vi "terminal point.vi"(2 "peaks/valleys":enum32{"Peaks", "Valleys"}(ring)=enum."Valleys", 3 "threshold":dbl caption="阈值" format="%0.2f", 4 "PD width":i32=3 caption="PD宽度" min=3, 5 "TDD filePath":path caption="TDD file Path") -> (0 "time low":dbl, 1 "time low index":dbl)   [LabVIEW 2011]
uses:
  <vilib>/Utility/file.llb/Read From Spreadsheet File (DBL).vi
  <vilib>/Analysis/NI_AAL_SigProc.lvlib
panel:
  out "XY图":cluster{"all rows":dbl[], "all rows":dbl[]}[](graph)
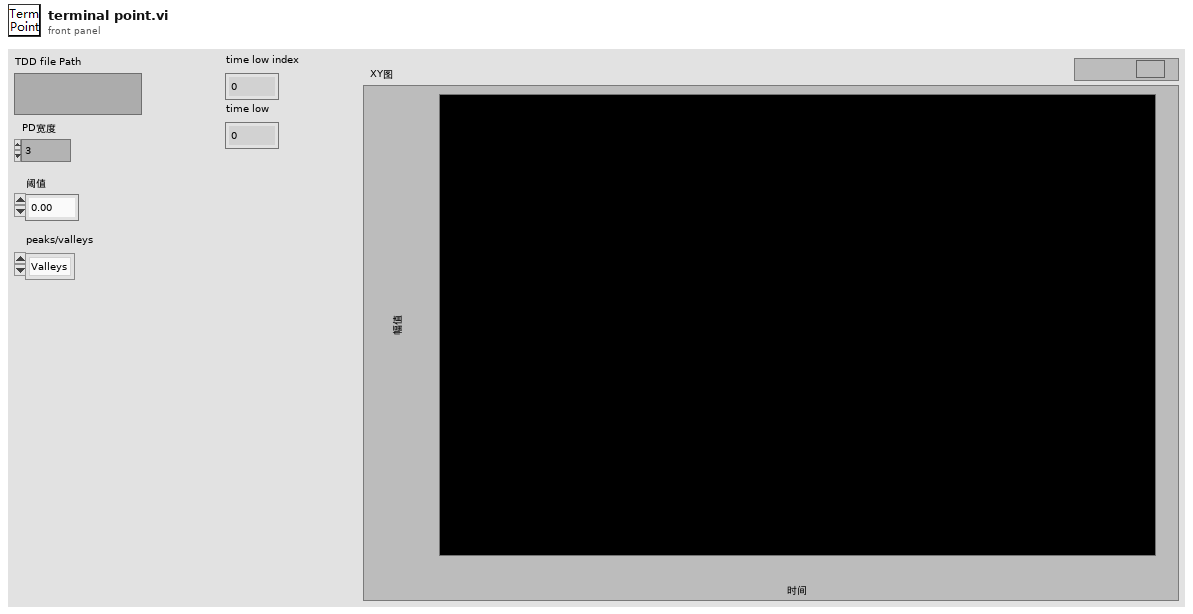
[diagram p1: front panel]
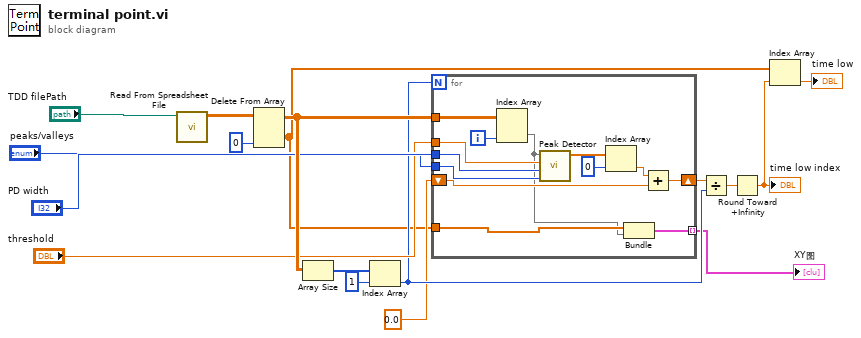
[diagram p0: block diagram]
diagram:
  n1 = call-poly <vilib>:"Read From Spreadsheet File.vi"("file path (dialog if empty)"="TDD filePath") -> ("all rows"=w15:dbl[][])  [unwired: 6 in, 4 out]
  n2 = Delete From Array(array=w15, index (col)=0 ("禁用的索引 (列)")) -> (deleted portion=w2:dbl[], array with subset deleted=w12:dbl[][])  [unwired: 2 in]
  n3 = Array Size(array=w12) -> (size(s)=w14:i32[])
  n4 = Index Array(array=w14, index=1 ("索引")) -> (element=w7:i32)
  n5 = for {
    N: w7 -> [_]
    tunnel: w12 -> [w30]
    tunnel: "PD width" -> [w28]
    tunnel: "peaks/valleys" -> [w27]
    tunnel: "threshold" -> [w26]
    shift-right: [w23] -> w8
    shift-left: 0.0 -> [w24]
    tunnel: w2 -> [w19]
    tunnel: [w20] -> w1 mode=indexing
    i -> [w29]
    n6 = Index Array(array=w30, index (col)=w29) -> (element=w18:dbl[])  [unwired: 1 in]
    n7 = call <vilib>:"Peak Detector.vi"("peaks/valleys"=w27, "width"=w28, "threshold"=w26, "X"=w18) -> ("Locations"=w25:dbl[])  [unwired: 3 in, 4 out]
    n8 = Index Array(array=w25, index=0 ("索引")) -> (element=w22:dbl)
    n9 = Bundle("all rows"=w19, "all rows"=w18) -> (w20:cluster{"all rows":dbl[], "all rows":dbl[]})  [unwired: 1 in]
    n10 = Add(x=w22, y=w24) -> (x+y=w23:dbl)
  }
  "XY图" <- w1
  n11 = Divide(x=w8, y=w7) -> (x/y=w6:dbl)
  n12 = Round Toward +Infinity(x=w6) -> (ceil(x): smallest int >= x=w5:dbl)
  "time low index" <- w5
  n13 = Index Array(array=w2, index=w5) -> (element=→"time low":dbl)
